vi "Backup_Client.vi"(1 "Check Updates on Server?":bool, 2 "Get all Server Files":bool, 3 "Months of History to backup":i32) -> (0 "error out":errorcluster)   [LabVIEW 2014]
uses:
  Anemometry/Anemometry Sub Vis/Globals/Preference_global.vi
  Anemometry/Anemometry Sub Vis/Globals/Constants_global.vi
panel:
  out "Currrently Working on":path
  out "Log of folder Done":T1(array[cluster])
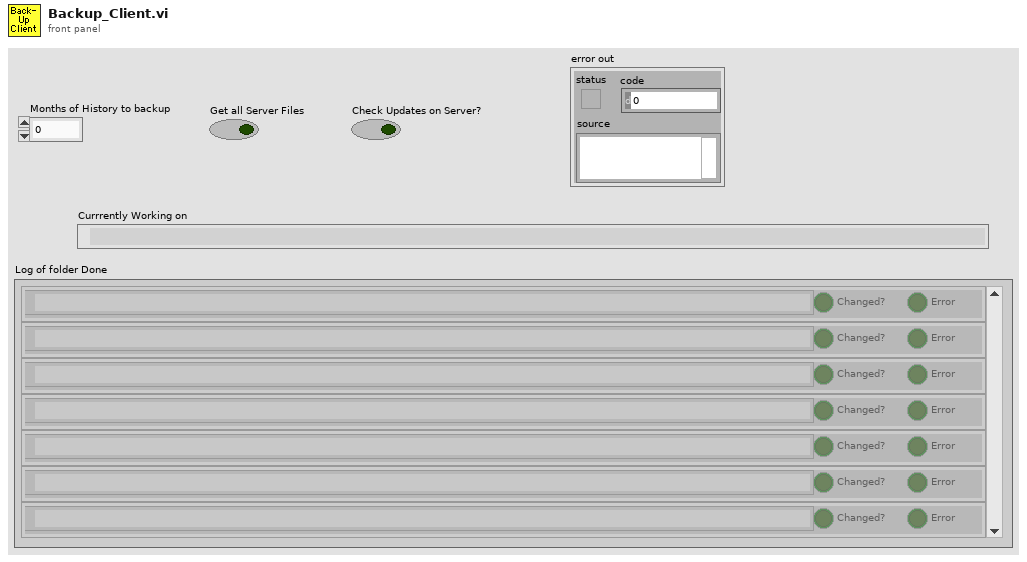
[diagram p1: front panel]
types:
  T1 = cluster{"Curnently on":path, "Changed?":bool, "Error":bool}[]
  T2 = typedef "EnFlo_Data_Folder_Setup.ctl" = string
  T3 = typedef "LVDateTimeRec.ctl" = cluster{"fractional second":dbl, "second":i32, "minute":i32, "hour":i32, "day of month":i32, "month":i32, "year":i32, "day of week":i32, "day of year":i32, "DST":i32}
  T4 = cluster{"Curnently on":path, "Changed?":bool, "Error":bool}
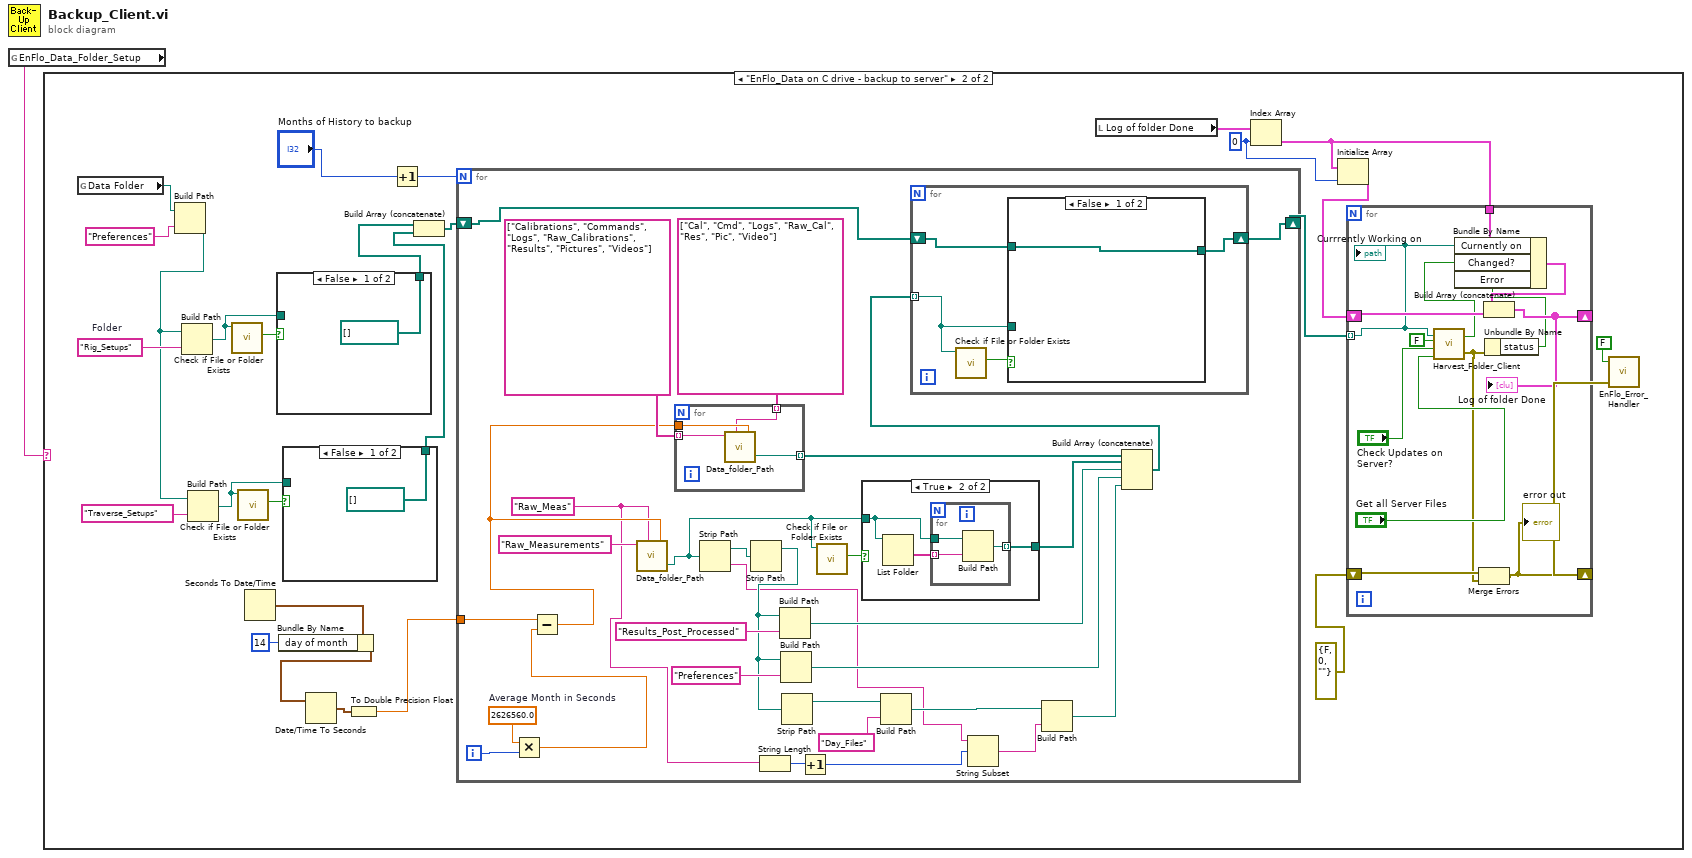
[diagram p0: block diagram]
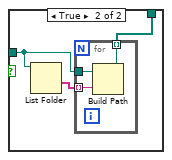
[diagram p3: hidden frame]
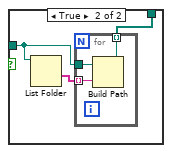
[diagram p4: hidden frame]
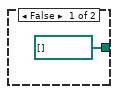
[diagram p5: hidden frame]
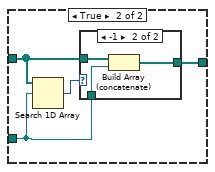
[diagram p6: hidden frame]
diagram:
  n1 = global read "Preference_global.vi" "EnFlo_Data_Folder_Setup"() -> (w1:T2)
  n2 = case shown="\"EnFlo_Data on C drive - backup to server\"" w1 {
    frame "No Match", Default {
    }
    frame "EnFlo_Data on C drive - backup to server" {
      w3 = 0 ("index")
      w12 = "Rig_Setups"  # Folder
      n3 = global read "Constants_global.vi" "Data Folder"() -> (w20:path)
      n4 = Build Path(base path=w20, name or relative path="Preferences") -> (appended path=w11:path)
      n5 = Build Path(base path=w11, name or relative path=w12) -> (appended path=w14:path)
      n6 = Build Path(base path=w11, name or relative path="Traverse_Setups") -> (appended path=w15:path)
      n7 = call <vilib>:"Check if File or Folder Exists.vi"("path"=w14) -> ("file or folder exists?"=w13:bool)  [unwired: 8 in, 2 out]
      n8 = call <vilib>:"Check if File or Folder Exists.vi"("path"=w15) -> ("file or folder exists?"=w16:bool)  [unwired: 8 in, 2 out]
      n9 = Seconds To Date/Time() -> (date time rec=w25:T3)  [unwired: 2 in]
      n10 = case shown="False" w13 {
        tunnel: [path[] [] w31] -> w9
        tunnel: w14 -> [_ w30]
        frame False {
        }
        frame True {
          n11 = List Folder(path=w30) -> (folder names=w32:string[])  [unwired: 3 in, 3 out]
          n12 = for {
            tunnel: w32 -> [w35] mode=indexing
            tunnel: w30 -> [w34]
            tunnel: [w33] -> w31 mode=indexing
            n13 = Build Path(base path=w34, name or relative path=w35) -> (appended path=w33:path)
          }
        }
      }
      n14 = Bundle By Name(cluster=w25, "day of month"=14) -> (w23:T3)
      n15 = case shown="False" w16 {
        tunnel: [path[] [] w38] -> w10
        tunnel: w15 -> [_ w37]
        frame False {
        }
        frame True {
          n16 = List Folder(path=w37) -> (folder names=w39:string[])  [unwired: 3 in, 3 out]
          n17 = for {
            tunnel: w39 -> [w42] mode=indexing
            tunnel: w37 -> [w41]
            tunnel: [w40] -> w38 mode=indexing
            n18 = Build Path(base path=w41, name or relative path=w42) -> (appended path=w40:path)
          }
        }
      }
      n19 = Date/Time To Seconds(2:w23) -> (0:w22:timestamp)  [unwired: 1 in]
      n20 = To Double Precision Float(number=w22) -> (double precision float=w26:dbl)
      n21 = Increment(x="Months of History to backup") -> (x+1=w28:i32)
      n22 = Build Array (concatenate)(w9, w10) -> (w18:path[])
      n23 = for {
        N: w28 -> [_]
        tunnel: w26 -> [w75]
        shift-right: [w70] -> w21
        shift-left: w18 -> [w71]
        i -> [w77]
        w60 = "Raw_Meas" ("Short_Name")
        w78 = 2626560.0  # Average Month in Seconds
        n24 = Multiply(x=w78, y=w77) -> (x*y=w76:dbl)
        n25 = Subtract(x=w75, y=w76) -> (x-y=w74:dbl)
        n26 = call "Data_folder_Path.vi"("Data Type"="Raw_Measurements", "Short_Name"=w60, "seconds"=w74) -> ("Data Folder"=w69:path)  [unwired: 3 in]
        n27 = for {
          tunnel: string[] ["Calibrations", "Commands", "Logs", "Raw_Calibrations", "Results", "Pictures", "Videos"] ("appended array") -> [w109] mode=indexing
          tunnel: [w108] -> w84 mode=indexing
          tunnel: w74 -> [w107]
          tunnel: string[] ["Cal", "Cmd", "Logs", "Raw_Cal", "Res", "Pic", "Video"] ("appended array") -> [w106] mode=indexing
          n28 = call "Data_folder_Path.vi"("Data Type"=w109, "Short_Name"=w106, "seconds"=w107) -> ("Data Folder"=w108:path)  [unwired: 3 in]
        }
        n29 = Strip Path(path=w69) -> (stripped path=w73:path, name=w57:string)
        n30 = Strip Path(path=w73) -> (stripped path=w66:path)  [unwired: 1 out]
        n31 = String Length(string=w60) -> (length=w59:i32)
        n32 = Build Path(base path=w66, name or relative path="Results_Post_Processed") -> (appended path=w80:path)
        n33 = Build Path(base path=w66, name or relative path="Preferences") -> (appended path=w67:path)
        n34 = Strip Path(path=w66) -> (stripped path=w65:path)  [unwired: 1 out]
        n35 = Increment(x=w59) -> (x+1=w58:i32)
        n36 = call <vilib>:"Check if File or Folder Exists.vi"("path"=w69) -> ("file or folder exists?"=w68:bool)  [unwired: 8 in, 2 out]
        n37 = case shown="True" w68 {
          tunnel: [path[] [] w88] -> w79
          tunnel: w69 -> [_ w87]
          frame False {
          }
          frame True {
            n38 = List Folder(path=w87) -> (folder names=w89:string[])  [unwired: 3 in, 3 out]
            n39 = for {
              tunnel: w89 -> [w92] mode=indexing
              tunnel: w87 -> [w91]
              tunnel: [w90] -> w88 mode=indexing
              n40 = Build Path(base path=w91, name or relative path=w92) -> (appended path=w90:path)
            }
          }
        }
        n41 = Build Path(base path=w65, name or relative path="Day_Files") -> (appended path=w63:path)
        n42 = String Subset(string=w57, offset (0)=w58) -> (substring=w56:string)  [unwired: 1 in]
        n43 = Build Path(base path=w63, name or relative path=w56) -> (appended path=w62:path)
        n44 = Build Array (concatenate)(w84, w79, w80, w67, w62) -> (w72:path[])
        n45 = for {
          shift-right: [w95] -> w70
          shift-left: w71 -> [w96]
          tunnel: w72 -> [w94] mode=indexing
          n46 = call <vilib>:"Check if File or Folder Exists.vi"("path"=w94) -> ("file or folder exists?"=w93:bool)  [unwired: 8 in, 2 out]
          n47 = case shown="False" w93 {
            tunnel: w96 -> [w97 w100]
            tunnel: w94 -> [_ w99]
            tunnel: [w97 w101] -> w95
            frame False {
            }
            frame True {
              n48 = Search 1D Array(1D array=w100, element=w99) -> (index of element=w98:i32)  [unwired: 1 in]
              n49 = case shown="-1" w98 {
                tunnel: w100 -> [w102 w105]
                tunnel: [w102 w104] -> w101
                tunnel: w99 -> [_ w103]
                frame 0, Default {
                }
                frame -1 {
                  n50 = Build Array (concatenate)(w105, w103) -> (w104:path[])
                }
              }
            }
          }
        }
      }
      n51 = local read "Log of folder Done"() -> (w5:T1)
      n52 = Index Array(array=w5, index=w3) -> (element=w4:T4)
      n53 = Initialize Array(w4, w3) -> (w2:T1)
      n54 = for {
        tunnel: w21 -> [w48] mode=indexing
        shift-right: [w46] -> w6
        shift-left: errorcluster {"status"=FALSE, "code"=0, "source"=""} ("error constant") -> [w52]
        shift-right: [w45] -> _
        shift-left: w2 -> [w51]
        tunnel: w4 -> [w50]
        n55 = call "Harvest_Folder_Client.vi"("Get all Server Files"="Get all Server Files", "Check Updates on Server?"="Check Updates on Server?", "Archive Files?"=FALSE, "Folder to Harvest"=w48) -> ("error out"=w44:errorcluster, "Folder contents changed?"=w49:bool)  [unwired: 2 out]
        n56 = Merge Errors(w52, w44) -> (w46:errorcluster)
        "error out" <- w46
        n57 = Unbundle By Name(w44) -> ("status"=w43:bool)
        n58 = Bundle By Name(cluster=w50, "Curnently on"=w48, "Changed?"=w49, "Error"=w43) -> (w47:T4)
        n59 = Build Array (concatenate)(w47, w51) -> (w45:T1)
        "Log of folder Done" <- w45
        "Currrently Working on" <- w48
      }
      n60 = call "EnFlo_Error_Handler.vi"("error in (no error)"=w6, "Dialog Box (T)"=FALSE) -> ()  [unwired: 1 in, 3 out]
    }
  }
